vi "SW_Load_frames_from_temp_XML_AA.vi"(2 "Error In":errorcluster, 3 "Input XML string":string) -> (0 "Error Out":errorcluster, 1 "Output array of data":string[][](array[string]))   [LabVIEW 2016]
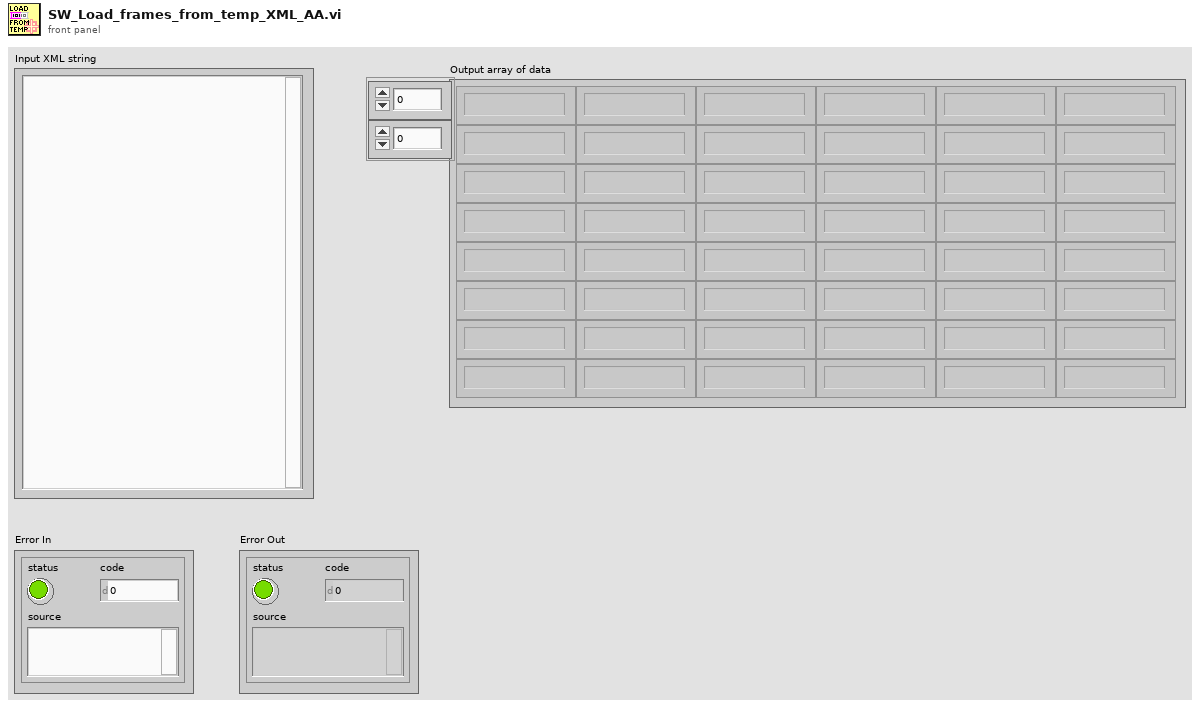
[diagram p1: front panel]
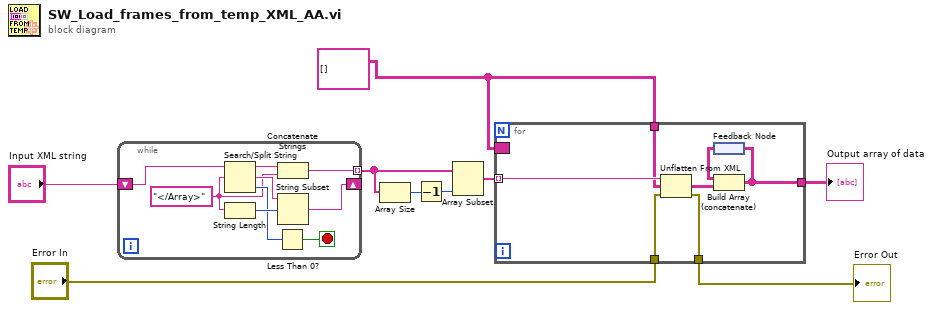
[diagram p0: block diagram]
diagram:
  w2 = string[][] []
  n1 = while {
    shift-right: [w15] -> _
    shift-left: "Input XML string" -> [w18]
    tunnel: [w11] -> w6 mode=indexing
    stop <- w13 stop-if-true
    w10 = "</Array>" ("search string/char (-)")
    n2 = Search/Split String(string=w18, search string/char (-)=w10) -> (substring before match=w12:string, match + rest of string=w16:string, offset of match=w14:i32)  [unwired: 1 in]
    n3 = String Length(string=w10) -> (length=w17:i32)
    n4 = Less Than 0?(x=w14) -> (x < 0?=w13:bool)
    n5 = Concatenate Strings(w12, w10) -> (w11:string)
    n6 = String Subset(string=w16, offset (0)=w17) -> (substring=w15:string)  [unwired: 1 in]
  }
  n7 = Array Size(array=w6) -> (size(s)=w7:i32)
  n8 = Decrement(x=w7) -> (x-1=w8:i32)
  n9 = Array Subset(array=w6, length=w8) -> (w9:string[])  [unwired: 1 in]
  n10 = for {
    tunnel: w9 -> [w25] mode=indexing
    tunnel: [w23] -> w1
    border: w2 -> [_]
    tunnel: w2 -> [w21]
    tunnel: "Error In" -> [w20]
    tunnel: [w19] -> w3
    n11 = Unflatten From XML(xml string=w25, type=w21, error in (no error)=w20) -> (value=w22:string[][], error out=w19:errorcluster)
    n12 = feedback #1() -> (w24:string[][])
    n13 = Build Array (concatenate)(w24, w22) -> (w23:string[][])
    n14 = feedback-in #1(w23) -> ()
  }
  "Error Out" <- w3
  "Output array of data" <- w1
